vi "Shoot2.vi"(8 "error in (no error)":errorcluster, 9 "Use Camera":bool, 10 "Auto Start":u32, 11 "Distance":dbl) -> (0 "error out":errorcluster)   [LabVIEW 2011]
uses:
  ShooterStates.ctl
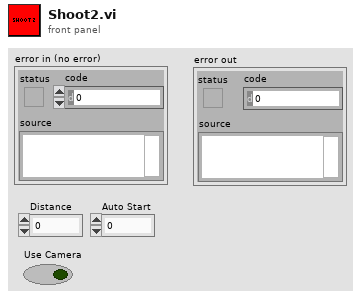
[diagram p1: front panel]
types:
  T1 = typedef "ShooterStates.ctl" = enum16{"Wait", "Aquire", "SpinUp", "Shoot", "Test"}
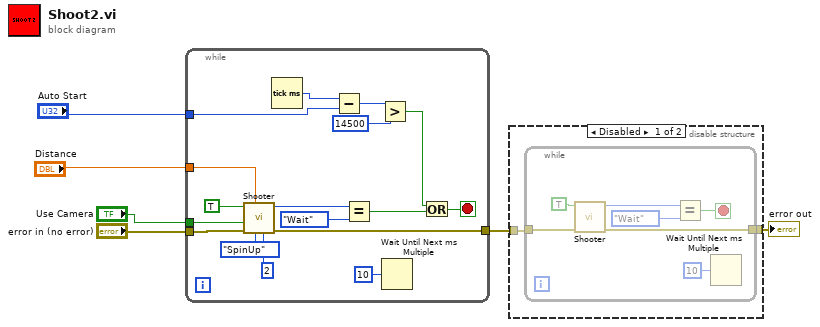
[diagram p0: block diagram]
diagram:
  n1 = while {
    tunnel: "error in (no error)" -> [w20]
    tunnel: [w19] -> w6
    tunnel: "Distance" -> [w17]
    tunnel: "Use Camera" -> [w16]
    tunnel: "Auto Start" -> [w12]
    stop <- w15 stop-if-true
    n2 = call "Shooter.vi"("Ball Count"=i8 2, "Aquire Fail Action"=ShooterStates."SpinUp", "Distance"=w17, "error in (no error)"=w20, "Use Camera"=w16, "Fire"=TRUE) -> ("error out"=w19:errorcluster, "Shooter State"=w22:T1)  [unwired: 4 in]
    n3 = Tick Count (ms)() -> (millisecond timer value=w13:u32)
    n4 = Subtract(x=w13, y=w12) -> (x-y=w11:u32)
    n5 = Equal?(x=w22, y=ShooterStates."Wait" ("Shooter State")) -> (x = y?=w14:bool)
    n6 = Greater?(x=w11, y=u32 14500) -> (0:w9:bool)
    n7 = Wait Until Next ms Multiple(millisecond multiple=u32 10) -> ()  [unwired: 1 out]
    n8 = Or(x=w9, y=w14) -> (x .or. y?=w15:bool)
  }
  n9 = disable-structure shown="Disabled" {
    disable-tunnel: w6 -> [w25 _]
    disable-tunnel: [w24 _] -> w5
    frame Disabled {
      n10 = while {
        tunnel: w25 -> [w28]
        tunnel: [w27] -> w24
        stop <- w29 stop-if-true
        n11 = call "Shooter.vi"("error in (no error)"=w28, "Fire"=TRUE) -> ("error out"=w27:errorcluster, "Shooter State"=w31:T1)  [unwired: 8 in]
        n12 = Equal?(x=w31, y=ShooterStates."Wait" ("Shooter State")) -> (x = y?=w29:bool)
        n13 = Wait Until Next ms Multiple(millisecond multiple=u32 10) -> ()  [unwired: 1 out]
      }
    }
    frame Enabled {
    }
  }
  "error out" <- w5
